vi "NewBackground.vi"(8 "error in (no error)":errorcluster, 11 "Snake in":refnum<class "Snake.lvclass">) -> (0 "error out":errorcluster, 3 "Snake out":refnum<class "Snake.lvclass">)   [LabVIEW 2019, in "RT_Game.lvlib" / "Snake.lvclass"]
uses:
  Snake.lvclass
  Game/TileCodes.ctl
  Snake.lvclass/Snake.ctl
  Game/Game.lvclass
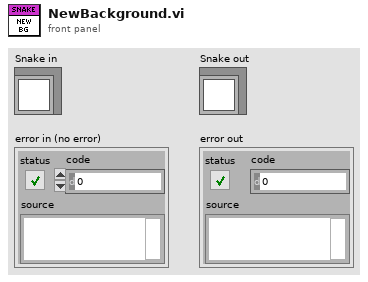
[diagram p1: front panel]
types:
  T1 = typedef "RT_Game.lvlib/Game.lvclass/TileCodes.ctl" = enum16{"line_vert", "line_hor", "line_rightup", "line_rightdown", "line_leftup", "line_leftdown", "bg1", "bg2", "bg3", "bg4", "bg5", "bg6", "bg7"}
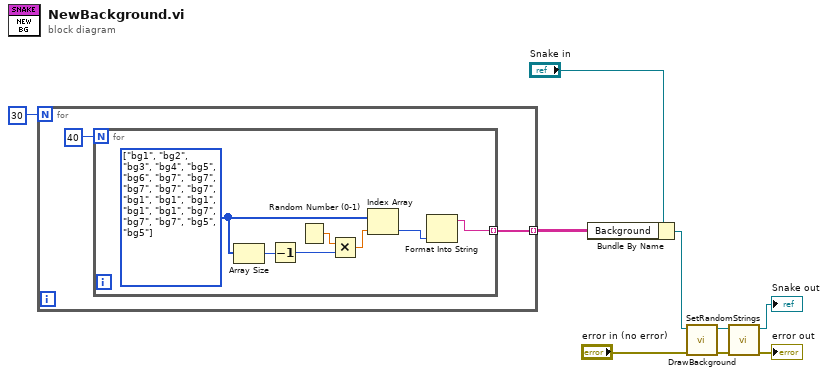
[diagram p0: block diagram]
diagram:
  n1 = for {
    N: 30 -> [_]
    tunnel: [w11] -> w9 mode=indexing
    n2 = for {
      N: 40 -> [_]
      tunnel: [w12] -> w11 mode=indexing
      w16 = T1[] [enum."bg1", enum."bg2", enum."bg3", enum."bg4", enum."bg5", enum."bg6", enum."bg7", enum."bg7", enum."bg7", enum."bg7", enum."bg7", enum."bg1", enum."bg1", enum."bg1", enum."bg1", enum."bg1", enum."bg7", enum."bg7", enum."bg7", enum."bg5", enum."bg5"] items=["line_vert", "line_hor", "line_rightup", "line_rightdown", "line_leftup", "line_leftdown", "bg1", "bg2", "bg3", "bg4", "bg5", "bg6", "bg7"] ("Array")
      n3 = Array Size(array=w16) -> (size(s)=w15:i32)
      n4 = Decrement(x=w15) -> (x-1=w14:i32)
      n5 = Random Number (0-1)() -> (number: 0 to 1=w18:dbl)
      n6 = Multiply(x=w18, y=w14) -> (x*y=w17:dbl)
      n7 = Index Array(array=w16, index=w17) -> (element=w13:T1)
      n8 = Format Into String(w13) -> (resulting string=w12:string)  [unwired: 3 in, 1 out]
    }
  }
  n9 = Bundle By Name(cluster="Snake in", "Background"=w9) -> (w4:refnum<class "Snake.lvclass">)
  n10 = call "DrawBackground.vi"("error in (no error)"="error in (no error)", "Snake in"=w4) -> ("error out"=w5:errorcluster, "Snake out"=w2:refnum<class "Snake.lvclass">)  [unwired: 8 in]
  n11 = call "SetRandomStrings.vi"("error in (no error)"=w5, "Snake in"=w2) -> ("error out"=→"error out":errorcluster, "Snake out"=→"Snake out":refnum<class "Snake.lvclass">)  [unwired: 8 in]
